vi "GT Get Lead Screw Comp Inner Value.vi"(6 "pCompValue":i32, 7 "pos":i32, 8 "error in (no error)":errorcluster caption="错误输入（无错误）", 9 "dir":i16, 10 "axis":i16, 11 "cardNum":i16) -> (0 "error out":errorcluster caption="错误输出", 3 "function return":i16, 4 "pCompValue out":i32)   [LabVIEW 2020, in "gts.lvlib"]
doc: "GT_API GT_GetLeadScrewCompInnerValue(short cardNum,short axis,short dir,long pos,long *pCompValue);"
uses:
  gts.lvlib
  dll/32bit/multi_card/gts.dll
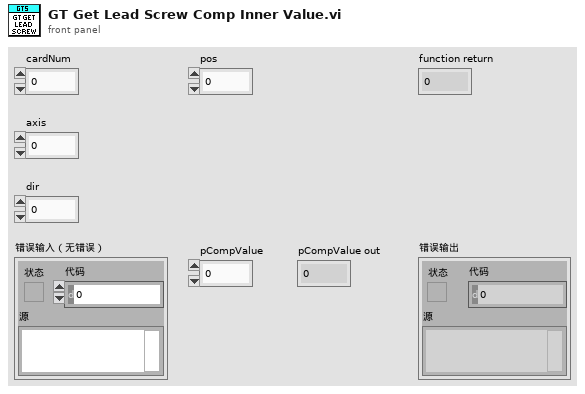
[diagram p1: front panel]
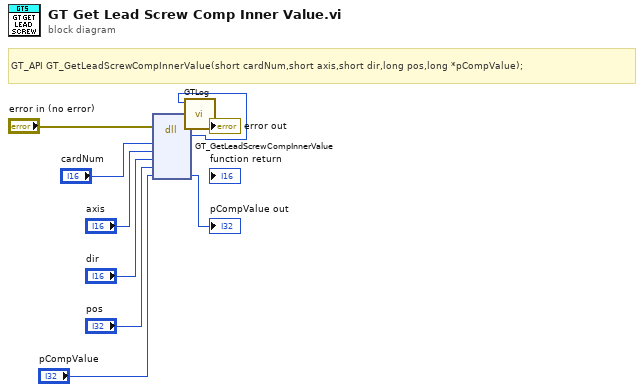
[diagram p0: block diagram]
diagram:
  # "GT_API GT_GetLeadScrewCompInnerValue(short cardNum,short axis,short dir,long pos,long *pCompValue);"
  n1 = dll-call lib="C:/1228/dll/32bit/multi_card/gts.dll" fn="GT_GetLeadScrewCompInnerValue"(error in="error in (no error)", "cardNum"="cardNum", "axis"="axis", "dir"="dir", "pos"="pos", "pCompValue"="pCompValue") -> (error out=w3:errorcluster, w1:i16, "pCompValue"=→"pCompValue out":i32)  [unwired: 6 in, 1 out]
  n2 = call "GTLog.vi"("error in (no error)"=w3, "Numeric"=w1) -> ("error out"=→"error out":errorcluster)  [unwired: 9 in]
